vi "SampleGetIDSingle.vi"() -> ()   [LabVIEW 2013]
panel:
  out "Identification":string
  out "error out":errorcluster
  out "DeviceKey Out":string
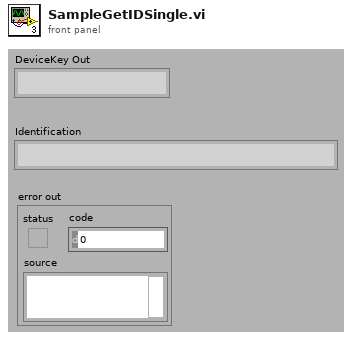
[diagram p1: front panel]
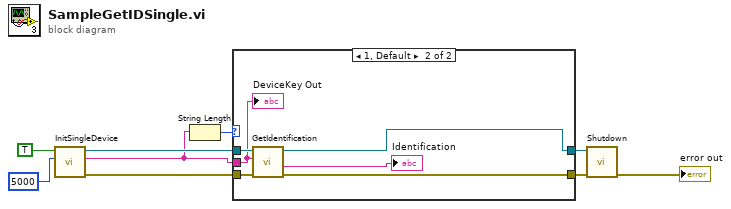
[diagram p0: block diagram]
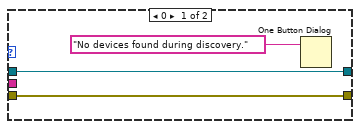
[diagram p2: hidden frame]
diagram:
  n1 = call "InitSingleDevice.vi"("msecDelayForDiscovery"=5000, "logging"=TRUE) -> ("error out"=w2:errorcluster, "DeviceKey Out"=w1:string, "CmdLib Out"=w3:refnum<k24>)  [unwired: 3 in]
  n2 = String Length(string=w1) -> (length=w6:i32)
  n3 = case shown="1, Default" w6 {
    tunnel: [w12 w17] -> w5
    tunnel: [w11 w16] -> w4
    tunnel: w3 -> [w12 w15]
    tunnel: w2 -> [w11 w14]
    tunnel: w1 -> [_ w13]
    frame 0 {
      n4 = One Button Dialog(message="No devices found during discovery.") -> ()  [unwired: 1 in, 1 out]
    }
    frame 1, Default {
      n5 = call "GetIdentification.vi"("error in (no error)"=w14, "DeviceKey In"=w13, "CmdLib In"=w15) -> ("error out"=w16:errorcluster, "Identification"=→"Identification":string, "CmdLib Out"=w17:refnum<k24>)  [unwired: 1 in, 1 out]
      "DeviceKey Out" <- w13
    }
  }
  n6 = call "Shutdown.vi"("error in (no error)"=w4, "CmdLib In"=w5) -> ("error out"=→"error out":errorcluster)  [unwired: 4 in, 1 out]
